vi "Create Operators and Aliases.vi"(8 "error in":errorcluster) -> (0 "error out":errorcluster, 4 "log":string)   [LabVIEW 2024]
uses:
  <vilib>/Plug-In SDKs/Clients/Metadata/Operator.ctl
  <vilib>/Plug-In SDKs/Clients/Metadata/Extension Value.ctl
  <vilib>/Plug-In SDKs/Clients/Metadata Store V1/Metadata Store Client.lvlibp/API/Metadata Store V1/Create Operator.vi
  <vilib>/Plug-In SDKs/Clients/Metadata Store V1/Metadata Store Client.lvlibp/API/Metadata Store V1/Create Alias (Metadata - Operator).vi
  <vilib>/Plug-In SDKs/Clients/Metadata Store V1/Metadata Store Client.lvlibp
  <vilib>/Plug-In SDKs/Clients/Metadata/NI Metadata Types.lvlib
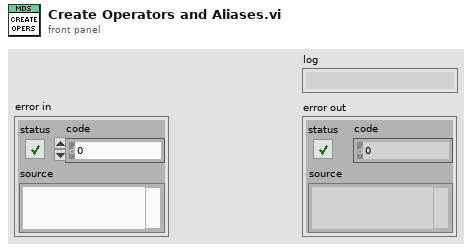
[diagram p1: front panel]
types:
  T1 = typedef "NI Metadata Types.lvlib/Operator.ctl" = cluster{"name":string, "role":string, "id":string, "link":string, "extension":T2[], "schema id":string}
  T2 = typedef "NI Metadata Types.lvlib/Extension Value.ctl" = cluster{"name":string, "value":string}
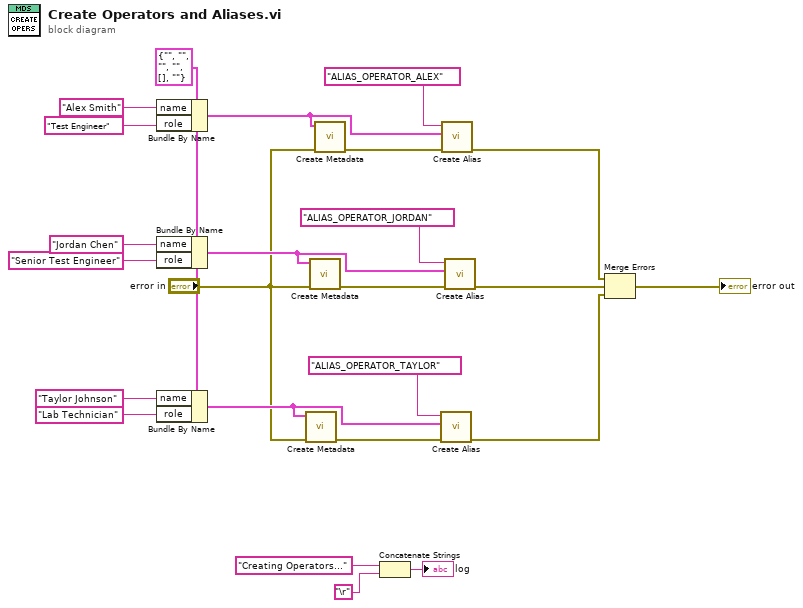
[diagram p0: block diagram]
diagram:
  w5 = T1 {"name"="", "role"="", "id"="", "link"="", "extension"=[], "schema id"=""} ("operator metadata")
  n1 = Bundle By Name(cluster=w5, "name"="Alex Smith" ("operator name"), "role"="Test Engineer") -> (w15:T1)
  n2 = Bundle By Name(cluster=w5, "name"="Jordan Chen" ("operator name"), "role"="Senior Test Engineer") -> (w20:T1)
  n3 = Bundle By Name(cluster=w5, "name"="Taylor Johnson" ("operator name"), "role"="Lab Technician") -> (w19:T1)
  n4 = call-poly <vilib>:"Create Metadata.vi"("error in"="error in", "operator metadata"=w19) -> ("error out"=w12:errorcluster)  [unwired: 8 in, 1 out]
  n5 = call-poly <vilib>:"Create Metadata.vi"("error in"="error in", "operator metadata"=w20) -> ("error out"=w13:errorcluster)  [unwired: 8 in, 1 out]
  n6 = call-poly <vilib>:"Create Metadata.vi"("error in"="error in", "operator metadata"=w15) -> ("error out"=w14:errorcluster)  [unwired: 8 in, 1 out]
  n7 = Concatenate Strings("Creating Operators..." ("role"), "\r") -> (→"log":string)
  n8 = call-poly <vilib>:"Create Alias.vi"("error in"=w12, "operator"=w19, "alias name"="ALIAS_OPERATOR_TAYLOR") -> ("error out"=w23:errorcluster)  [unwired: 7 in, 1 out]
  n9 = call-poly <vilib>:"Create Alias.vi"("error in"=w14, "operator"=w15, "alias name"="ALIAS_OPERATOR_ALEX") -> ("error out"=w21:errorcluster)  [unwired: 7 in, 1 out]
  n10 = call-poly <vilib>:"Create Alias.vi"("error in"=w13, "operator"=w20, "alias name"="ALIAS_OPERATOR_JORDAN") -> ("error out"=w22:errorcluster)  [unwired: 7 in, 1 out]
  n11 = Merge Errors(w21, w22, w23) -> (→"error out":errorcluster)
